vi "CRYWindow WAIT DataView.vi"(10 "vi reference":refnum<vi>, 11 "sAction":string) -> (1 "sData_Out":string)   [LabVIEW 2013]
panel:
  # "Wait until DataView Loading and Closing."
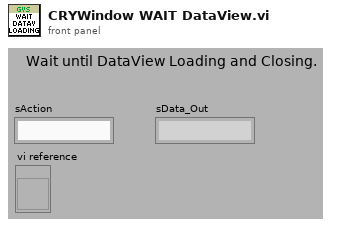
[diagram p1: front panel]
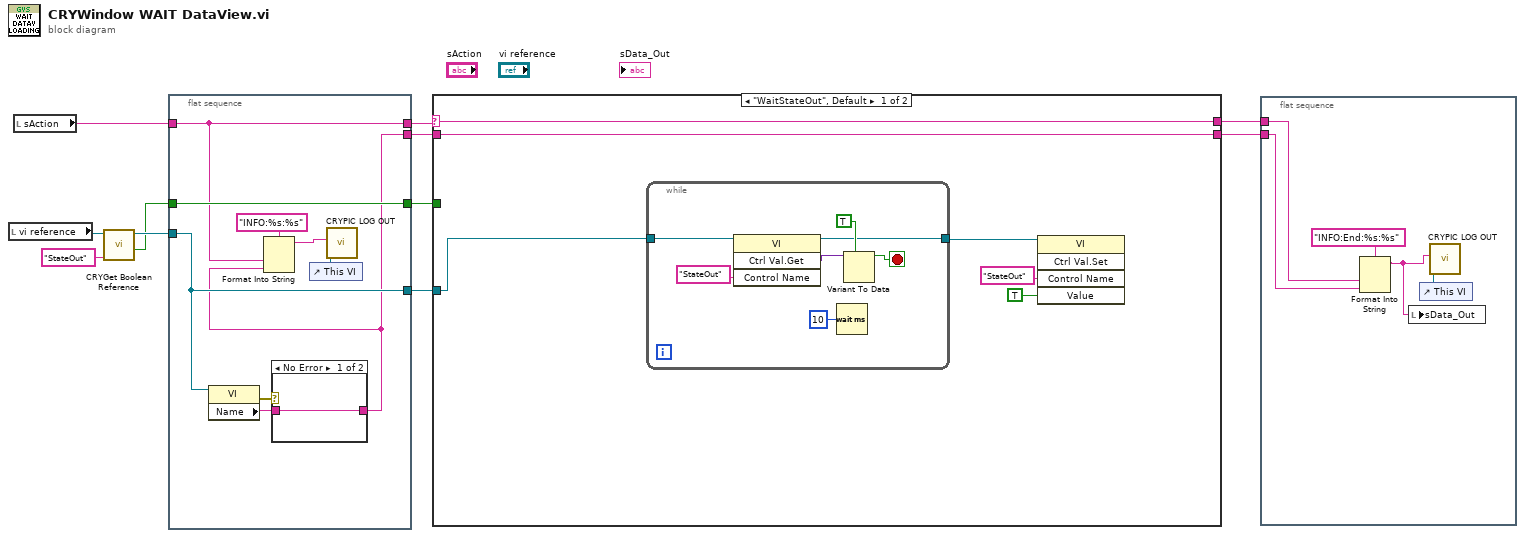
[diagram p0: block diagram]
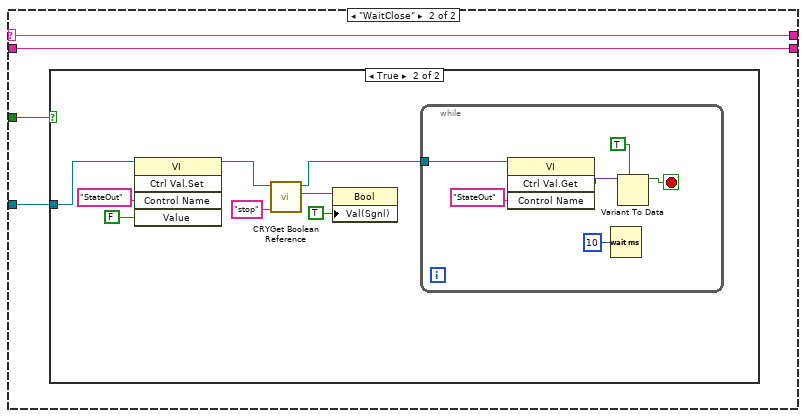
[diagram p2: hidden frame]
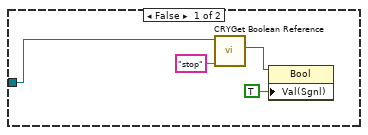
[diagram p3: hidden frame]
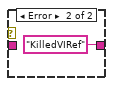
[diagram p4: hidden frame]
diagram:
  n1 = local read "vi reference"() -> (w6:refnum<vi>)
  n2 = local read "sAction"() -> (w5:string)
  n3 = call "CRYGet Boolean Reference.vi"("Label Name"="StateOut", "VI Refnum"=w6) -> ("Exist?"=w9:bool, "VI Refnum Out"=w10:refnum<vi>)  [unwired: 7 in, 1 out]
  n4 = flat-sequence {
    tunnel: [w16] -> w8
    tunnel: w10 -> [w16]
    tunnel: [w20] -> w7
    tunnel: w9 -> [w20]
    tunnel: w5 -> [w15]
    tunnel: [w15] -> w4
    tunnel: [w14] -> w2
    frame #0 {
      n5 = property class="VI"(reference=w16) -> (error out=w18:errorcluster, "Name"=w17:string)  [unwired: 1 in, 1 out]
      n6 = case shown="No Error" w18 {
        tunnel: w17 -> [w21 _]
        tunnel: [w21 "KilledVIRef" ("sAction")] -> w14
        frame No Error {
        }
        frame Error {
        }
      }
      n7 = Format Into String(format string="INFO:%s:%s" ("string"), w15, w14) -> (resulting string=w12:string)  [unwired: 2 in, 1 out]
      n8 = control-ref of="This VI"() -> (w13:refnum<vi>)
      n9 = call "CRYPIC LOG OUT.vi"("pVIRef"=w13, "sData"=w12) -> ()  [unwired: 10 in]
    }
  }
  n10 = case shown="\"WaitStateOut\", Default" w4 {
    selector: w4 -> [w28 w37]
    tunnel: w8 -> [w27 w39]
    tunnel: w7 -> [_ w38]
    tunnel: [w28 w37] -> w3
    tunnel: w2 -> [w26 w36]
    tunnel: [w26 w36] -> w1
    frame "WaitStateOut", Default {
      n11 = while {
        tunnel: w27 -> [w34]
        tunnel: [w29] -> w23
        stop <- w31 stop-if-true
        n12 = invoke class="VI" method="Ctrl Val.Get"(reference=w34, "Control Name"="StateOut") -> (reference out=w29:refnum<vi>, "Get Control Value Variant"=w33:variant)  [unwired: 2 in, 2 out]
        n13 = Wait (ms)(milliseconds to wait=u32 10) -> ()  [unwired: 1 out]
        n14 = Variant To Data(type=TRUE, Variant=w33) -> (data=w31:bool)  [unwired: 1 in, 1 out]
      }
      n15 = invoke class="VI" method="Ctrl Val.Set"(reference=w23, "Control Name"="StateOut", "Value"=TRUE) -> ()  [unwired: 2 in, 5 out]
    }
    frame "WaitClose" {
      n16 = case shown="True" w38 {
        tunnel: w39 -> [w40 w44]
        frame False {
          n17 = call "CRYGet Boolean Reference.vi"("Label Name"="stop", "VI Refnum"=w40) -> ("Boolean Ref"=w43:refnum<vi>)  [unwired: 7 in, 2 out]
          n18 = property class="Bool"(reference=w43, "Val(Sgnl)"=TRUE) -> ()  [unwired: 1 in, 2 out]
        }
        frame True {
          n19 = invoke class="VI" method="Ctrl Val.Set"(reference=w44, "Control Name"="StateOut", "Value"=FALSE) -> (reference out=w46:refnum<vi>)  [unwired: 2 in, 4 out]
          n20 = call "CRYGet Boolean Reference.vi"("Label Name"="stop", "VI Refnum"=w46) -> ("Boolean Ref"=w49:refnum<vi>, "VI Refnum Out"=w45:refnum<vi>)  [unwired: 7 in, 1 out]
          n21 = property class="Bool"(reference=w49, "Val(Sgnl)"=TRUE) -> ()  [unwired: 1 in, 2 out]
          n22 = while {
            tunnel: w45 -> [w56]
            stop <- w53 stop-if-true
            n23 = invoke class="VI" method="Ctrl Val.Get"(reference=w56, "Control Name"="StateOut") -> ("Get Control Value Variant"=w55:variant)  [unwired: 2 in, 3 out]
            n24 = Wait (ms)(milliseconds to wait=u32 10) -> ()  [unwired: 1 out]
            n25 = Variant To Data(type=TRUE, Variant=w55) -> (data=w53:bool)  [unwired: 1 in, 1 out]
          }
        }
      }
    }
  }
  n26 = flat-sequence {
    tunnel: w3 -> [w61]
    tunnel: w1 -> [w60]
    frame #0 {
      n27 = Format Into String(format string="INFO:End:%s:%s" ("string"), w61, w60) -> (resulting string=w58:string)  [unwired: 2 in, 1 out]
      n28 = local write "sData_Out"(w58) -> ()
      n29 = control-ref of="This VI"() -> (w59:refnum<vi>)
      n30 = call "CRYPIC LOG OUT.vi"("pVIRef"=w59, "sData"=w58) -> ()  [unwired: 10 in]
    }
  }
